vi "TCS_Stream.vi"() -> ()   [LabVIEW 2018]
uses:
  Stream/Stream.lvclass
  RxTx/RxTx.lvclass
  Stream/Stream.lvclass/Stream.ctl
panel:
  in  "RxTx.lvclass 2":refnum<class "RxTx.lvclass">
  in  "Stream.lvclass 2":refnum<class "Stream.lvclass">
  in  "RxTx.lvclass":refnum<class "RxTx.lvclass">
  in  "Stream.lvclass":refnum<class "Stream.lvclass">
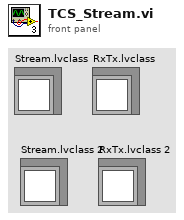
[diagram p1: front panel]
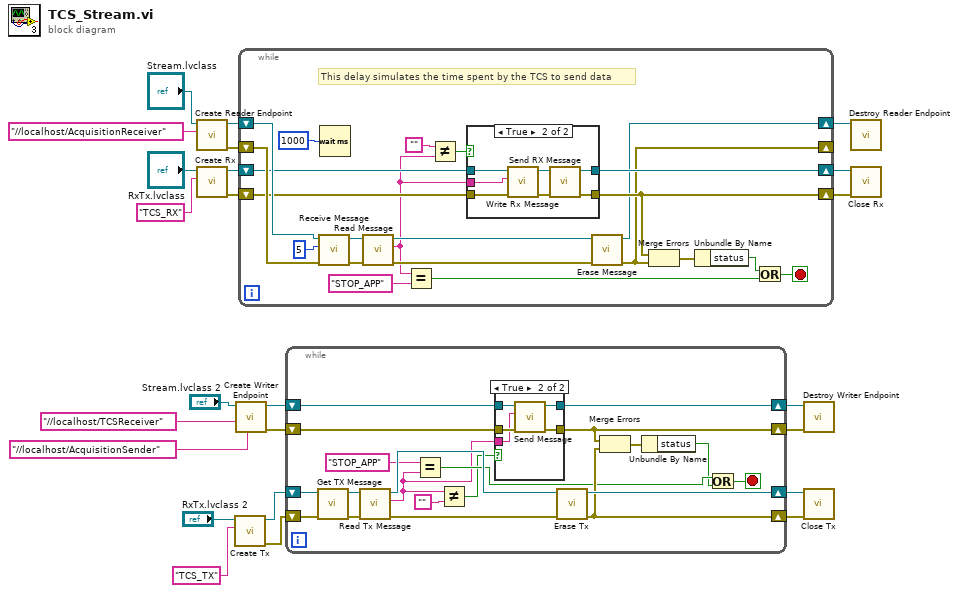
[diagram p0: block diagram]
diagram:
  n1 = call "Create Reader Endpoint.vi"("reader name"="//localhost/AcquisitionReceiver", "Stream in"="Stream.lvclass") -> ("error out"=w22:errorcluster, "Stream out"=w23:refnum<class "Stream.lvclass">)  [unwired: 8 in]
  n2 = call "Create Rx.vi"("Reader Name"="TCS_RX", "RxTx in"="RxTx.lvclass") -> ("error out"=w17:errorcluster, "RxTx out"=w18:refnum<class "RxTx.lvclass">)  [unwired: 8 in]
  n3 = call "Create Tx.vi"("Writer Name"="TCS_TX" ("Reader Name"), "RxTx in"="RxTx.lvclass 2") -> ("error out"=w11:errorcluster, "RxTx out"=w12:refnum<class "RxTx.lvclass">)  [unwired: 8 in]
  n4 = call "Create Writer Endpoint.vi"("writer name"="//localhost/AcquisitionSender" ("reader name"), "reader name"="//localhost/TCSReceiver", "Stream in"="Stream.lvclass 2") -> ("error out"=w5:errorcluster, "Stream out"=w7:refnum<class "Stream.lvclass">)  [unwired: 7 in]
  n5 = while {
    shift-right: [w31] -> _
    shift-left: w22 -> [w45]
    shift-right: [w34] -> w21
    shift-left: w23 -> [w46]
    shift-right: [w38] -> w15
    shift-left: w17 -> [w42]
    shift-right: [w40] -> w16
    shift-left: w18 -> [w41]
    stop <- w28 stop-if-true
    # "This delay simulates the time spent by the TCS to send data"
    n6 = call "Receive Message.vi"("error in (no error)"=w45, "timeout ms"=5, "Stream in"=w46) -> ("error out"=w43:errorcluster, "Stream out"=w44:refnum<class "Stream.lvclass">)  [unwired: 7 in]
    n7 = Wait (ms)(milliseconds to wait=u32 1000) -> ()  [unwired: 1 out]
    n8 = call "Read Message.vi"("error in (no error)"=w43, "Stream in"=w44) -> ("error out"=w33:errorcluster, "Message"=w30:string, "Stream out"=w32:refnum<class "Stream.lvclass">)  [unwired: 7 in]
    n9 = Equal?(x=w30, y="STOP_APP" ("reader name")) -> (x = y?=w26:bool)
    n10 = Not Equal?(x="", y=w30) -> (x != y?=w35:bool)
    n11 = case shown="True" w35 {
      tunnel: w42 -> [w47 w53]
      tunnel: w41 -> [w48 w52]
      tunnel: w30 -> [_ w51]
      tunnel: [w48 w50] -> w40
      tunnel: [w47 w49] -> w38
      frame False {
      }
      frame True {
        n12 = call "Write Rx Message.vi"("error in (no error)"=w53, "Rx Message"=w51, "RxTx in"=w52) -> ("error out"=w54:errorcluster, "RxTx out"=w55:refnum<class "RxTx.lvclass">)  [unwired: 7 in]
        n13 = call "Send RX Message.vi"("error in (no error)"=w54, "RxTx in"=w55) -> ("error out"=w49:errorcluster, "RxTx out"=w50:refnum<class "RxTx.lvclass">)  [unwired: 8 in]
      }
    }
    n14 = call "Erase Message.vi"("error in (no error)"=w33, "Stream in"=w32) -> ("error out"=w31:errorcluster, "Stream out"=w34:refnum<class "Stream.lvclass">)  [unwired: 8 in]
    n15 = Merge Errors(w38, w31) -> (w39:errorcluster)
    n16 = Unbundle By Name(w39) -> ("status"=w27:bool)
    n17 = Or(x=w27, y=w26) -> (x .or. y?=w28:bool)
  }
  n18 = while {
    shift-right: [w67] -> w4
    shift-left: w5 -> [w69]
    shift-right: [w68] -> w13
    shift-left: w7 -> [w70]
    shift-right: [w62] -> w8
    shift-left: w11 -> [w71]
    shift-right: [w64] -> w9
    shift-left: w12 -> [w72]
    stop <- w59 stop-if-true
    n19 = call "Get TX Message.vi"("error in (no error)"=w71, "RxTx in"=w72) -> ("error out"=w74:errorcluster, "RxTx out"=w73:refnum<class "RxTx.lvclass">)  [unwired: 8 in]
    n20 = call "Read Tx Message.vi"("error in (no error)"=w74, "RxTx in"=w73) -> ("error out"=w63:errorcluster, "Tx Message"=w57:string, "RxTx out"=w65:refnum<class "RxTx.lvclass">)  [unwired: 7 in]
    n21 = Equal?(x="STOP_APP", y=w57) -> (x = y?=w61:bool)
    n22 = Not Equal?(x=w57, y="") -> (x != y?=w56:bool)
    n23 = case shown="True" w56 {
      tunnel: w70 -> [w77 w82]
      tunnel: w69 -> [w76 w81]
      tunnel: [w77 w80] -> w68
      tunnel: w57 -> [_ w79]
      tunnel: [w76 w78] -> w67
      frame False {
      }
      frame True {
        n24 = call "Send Message.vi"("error in (no error)"=w81, "Message"=w79, "Stream in"=w82) -> ("error out"=w78:errorcluster, "Stream out"=w80:refnum<class "Stream.lvclass">)  [unwired: 7 in]
      }
    }
    n25 = call "Erase Tx.vi"("error in (no error)"=w63, "RxTx in"=w65) -> ("error out"=w62:errorcluster, "RxTx out"=w64:refnum<class "RxTx.lvclass">)  [unwired: 8 in]
    n26 = Merge Errors(w67, w62) -> (w75:errorcluster)
    n27 = Unbundle By Name(w75) -> ("status"=w60:bool)
    n28 = Or(x=w61, y=w60) -> (x .or. y?=w59:bool)
  }
  n29 = call "Destroy Writer Endpoint.vi"("error in (no error)"=w4, "Stream in"=w13) -> ()  [unwired: 8 in, 2 out]
  n30 = call "Close Tx.vi"("error in (no error)"=w8, "RxTx in"=w9) -> ()  [unwired: 8 in, 2 out]
  n31 = call "Destroy Reader Endpoint.vi"("Stream in"=w21) -> ()  [unwired: 9 in, 2 out]
  n32 = call "Close Rx.vi"("error in (no error)"=w15, "RxTx in"=w16) -> ()  [unwired: 8 in, 2 out]
